vi "SubVi_Conversor.vi"(11 "Entrada_U16":u16) -> (2 "Factor_de_potencia":dbl, 3 "Dato":dbl)   [LabVIEW 2017, in "Lib_Maestro_Ingen.lvlib"]
uses:
  Lib_Maestro_Ingen.lvlib
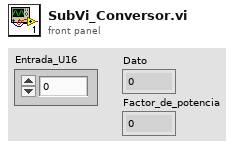
[diagram p1: front panel]
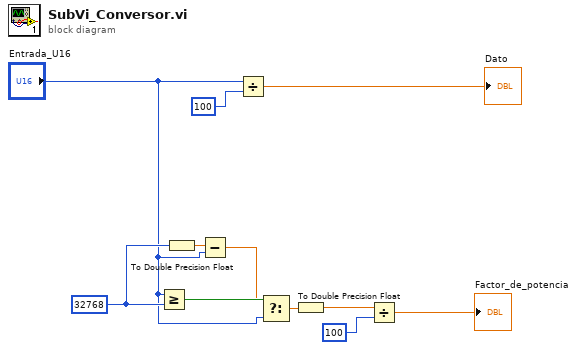
[diagram p0: block diagram]
diagram:
  w2 = u16 32768 ("y")
  n1 = Greater Or Equal?(x="Entrada_U16", y=w2) -> (x >= y?=w8:bool)
  n2 = To Double Precision Float(number=w2) -> (double precision float=w3:dbl)
  n3 = Subtract(x=w3, y="Entrada_U16") -> (x-y=w4:dbl)
  n4 = Divide(x="Entrada_U16", y=u16 100) -> (x/y=→"Dato":dbl)
  n5 = Select(t=w4, s=w8, f="Entrada_U16") -> (s? t:f=w7:dbl)
  n6 = To Double Precision Float(number=w7) -> (double precision float=w6:dbl)
  n7 = Divide(x=w6, y=u16 100) -> (x/y=→"Factor_de_potencia":dbl)
